vi "2 - 参数计算.vi"(8 "error in (no error)":errorcluster caption="错误输入（无错误）", 10 "采集信号输入":waveform(dbl)[](array[waveform]), 11 "显示控件引用输入":T1) -> (0 "error out":errorcluster caption="错误输出")   [LabVIEW 2019]
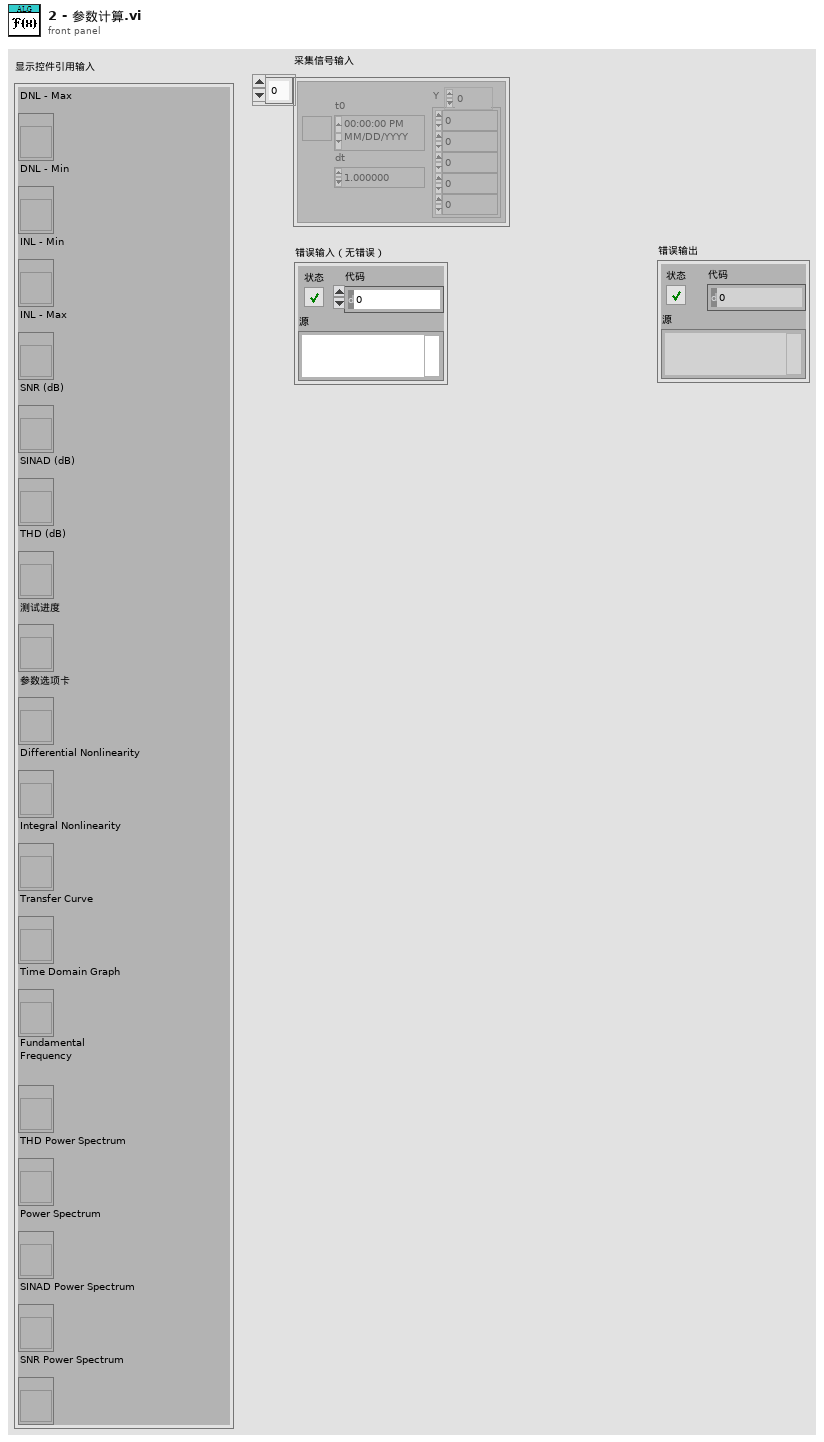
[diagram p1: front panel]
types:
  T1 = cluster{"DNL - Max":refnum<vi>, "DNL - Min":refnum<vi>, "INL - Min":refnum<vi>, "INL - Max":refnum<vi>, "SNR (dB)":refnum<vi>, "SINAD (dB)":refnum<vi>, "THD (dB)":refnum<vi>, "测试进度":refnum<vi>, "参数选项卡":refnum<vi>, "Differential Nonlinearity":refnum<vi>, "Integral Nonlinearity":refnum<vi>, "Transfer Curve":refnum<vi>, "Time Domain Graph":refnum<vi>, "Fundamental\nFrequency":refnum<vi>, "THD Power Spectrum":refnum<vi>, "Power Spectrum":refnum<vi>, "SINAD Power Spectrum":refnum<vi>, "SNR Power Spectrum":refnum<vi>}
  T2 = enum8{"Enabled", "Disabled", "Disabled and Grayed Out"}
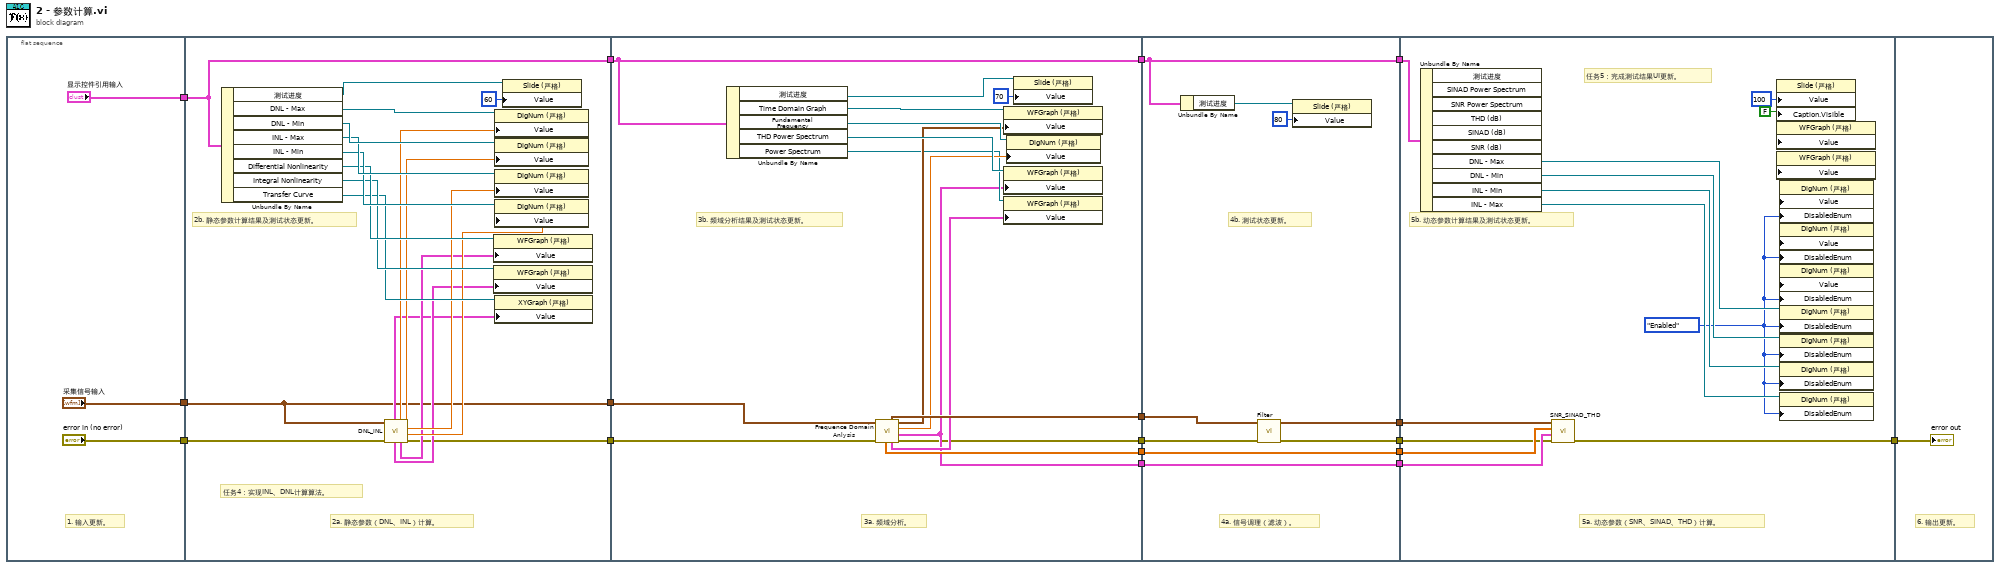
[diagram p0: block diagram]
diagram:
  n1 = flat-sequence {
    tunnel: ["采集信号输入"] -> w17
    tunnel: ["显示控件引用输入"] -> w16
    tunnel: ["error in (no error)"] -> w5
    tunnel: w17 -> [w23]
    tunnel: w16 -> [w24]
    tunnel: [w23] -> w15
    tunnel: [w24] -> w14
    tunnel: w5 -> [w22]
    tunnel: [w21] -> w4
    tunnel: w15 -> [w56]
    tunnel: w14 -> [w46]
    tunnel: [w55] -> w13
    tunnel: [w43] -> w12
    tunnel: [w54] -> w11
    tunnel: [w46] -> w10
    tunnel: w4 -> [w42]
    tunnel: [w41] -> w3
    tunnel: w13 -> [w63]
    tunnel: w12 -> [w65]
    tunnel: w11 -> [w64]
    tunnel: w10 -> [w59]
    tunnel: [w65] -> w9
    tunnel: [w64] -> w8
    tunnel: [w62] -> w7
    tunnel: [w59] -> w6
    tunnel: w3 -> [w58]
    tunnel: [w57] -> w2
    tunnel: w9 -> [w78]
    tunnel: w8 -> [w76]
    tunnel: w7 -> [w77]
    tunnel: w6 -> [w75]
    tunnel: w2 -> [w72]
    tunnel: [w71] -> w1
    tunnel: w1 -> [w79]
    frame #0 {
      # "1. 输入更新。"
    }
    frame #1 {
      # "任务4：实现INL、DNL计算算法。"
      # "2b. 静态参数计算结果及测试状态更新。"
      # "2a. 静态参数（DNL、INL）计算。"
      n2 = Unbundle By Name(w24) -> ("测试进度"=w26:refnum<vi>, "DNL - Max"=w40:refnum<vi>, "DNL - Min"=w39:refnum<vi>, "INL - Max"=w38:refnum<vi>, "INL - Min"=w37:refnum<vi>, "Differential Nonlinearity"=w36:refnum<vi>, "Integral Nonlinearity"=w35:refnum<vi>, "Transfer Curve"=w34:refnum<vi>)
      n3 = call "DNL_INL.vi"("error in (no error)"=w22, "采集信号输入"=w23) -> ("error out"=w21:errorcluster, "INL - Min"=w30:ext, "INL - Max"=w31:ext, "DNL - Min"=w32:dbl, "DNL"=w29:cluster{i32, i32, "Y[i]=X[i]*a+b":dbl[]}, "DNL - Max"=w33:dbl, "INL"=w28:cluster{dbl, i32, ext[]}, "Transfer Curve"=w27:cluster{dbl[], i32[]}[])  [unwired: 2 in]
      n4 = property class="WFGraph (严格)"(reference=w36, "Value"=w29) -> ()  [unwired: 1 in, 2 out]
      n5 = property class="WFGraph (严格)"(reference=w35, "Value"=w28) -> ()  [unwired: 1 in, 2 out]
      n6 = property class="DigNum (严格)"(reference=w40, "Value"=w33) -> ()  [unwired: 1 in, 2 out]
      n7 = property class="DigNum (严格)"(reference=w39, "Value"=w32) -> ()  [unwired: 1 in, 2 out]
      n8 = property class="DigNum (严格)"(reference=w38, "Value"=w31) -> ()  [unwired: 1 in, 2 out]
      n9 = property class="DigNum (严格)"(reference=w37, "Value"=w30) -> ()  [unwired: 1 in, 2 out]
      n10 = property class="XYGraph (严格)"(reference=w34, "Value"=w27) -> ()  [unwired: 1 in, 2 out]
      n11 = property class="Slide (严格)"(reference=w26, "Value"=u8 60 ("值")) -> ()  [unwired: 1 in, 2 out]
    }
    frame #2 {
      # "3b. 频域分析结果及测试状态更新。"
      # "3a. 频域分析。"
      n12 = Unbundle By Name(w46) -> ("测试进度"=w53:refnum<vi>, "Time Domain Graph"=w51:refnum<vi>, "Fundamental\nFrequency"=w50:refnum<vi>, "THD Power Spectrum"=w49:refnum<vi>, "Power Spectrum"=w45:refnum<vi>)
      n13 = call "Frequence Domain Anlysis.vi"("error in (no error)"=w42, "采集信号输入"=w56) -> ("error out"=w41:errorcluster, "THD Power Spectrum"=w43:cluster{"f0":dbl, "df":dbl, "magnitude":dbl[]}[], "detected fundamental frequency"=w47:dbl, "S-Waveform Out"=w48:waveform(dbl), "power spectrum"=w44:cluster{"f0":dbl, "df":dbl, "magnitude":dbl[]}, "O-Waveform"=w55:waveform(dbl), "Harmonics Data Out"=w54:dbl[])  [unwired: 3 in]
      n14 = property class="WFGraph (严格)"(reference=w51, "Value"=w48) -> ()  [unwired: 1 in, 2 out]
      n15 = property class="WFGraph (严格)"(reference=w49, "Value"=w43) -> ()  [unwired: 1 in, 2 out]
      n16 = property class="WFGraph (严格)"(reference=w45, "Value"=w44) -> ()  [unwired: 1 in, 2 out]
      n17 = property class="DigNum (严格)"(reference=w50, "Value"=w47) -> ()  [unwired: 1 in, 2 out]
      n18 = property class="Slide (严格)"(reference=w53, "Value"=u8 70 ("值")) -> ()  [unwired: 1 in, 2 out]
    }
    frame #3 {
      # "4b. 测试状态更新。"
      # "4a. 信号调理（滤波）。"
      n19 = Unbundle By Name(w59) -> ("测试进度"=w61:refnum<vi>)
      n20 = call "Filter.vi"("error in (no error)"=w58, "O-Waveform输入"=w63) -> ("error out"=w57:errorcluster, "F_Waveform输出"=w62:waveform(dbl))  [unwired: 8 in]
      n21 = property class="Slide (严格)"(reference=w61, "Value"=u8 80 ("值")) -> ()  [unwired: 1 in, 2 out]
    }
    frame #4 {
      w66 = T2."Enabled" ("禁用")
      # "任务5：完成测试结果UI更新。"
      # "5b. 动态参数计算结果及测试状态更新。"
      # "5a. 动态参数（SNR、SINAD、THD）计算。"
      n22 = Unbundle By Name(w75) -> ("DNL - Max"=w67:refnum<vi>, "DNL - Min"=w68:refnum<vi>, "INL - Min"=w69:refnum<vi>, "INL - Max"=w70:refnum<vi>)  [unwired: 6 out]
      n23 = call "SNR_SINAD_THD.vi"("error in (no error)"=w72, "THD Power Spectrum"=w78, "Harmonics Data Out"=w76, "F_Waveform输入"=w77) -> ("error out"=w71:errorcluster)  [unwired: 2 in, 5 out]
      n24 = property class="Slide (严格)"("Value"=u8 100 ("值"), "Caption.Visible"=FALSE ("标题.可见")) -> ()  [unwired: 2 in, 2 out]
      n25 = property class="WFGraph (严格)" props=["Value"]() -> ()  [unwired: 3 in, 2 out]
      n26 = property class="WFGraph (严格)" props=["Value"]() -> ()  [unwired: 3 in, 2 out]
      n27 = property class="DigNum (严格)" props=["Value", "DisabledEnum"]("DisabledEnum"=w66) -> ()  [unwired: 3 in, 2 out]
      n28 = property class="DigNum (严格)" props=["Value", "DisabledEnum"]("DisabledEnum"=w66) -> ()  [unwired: 3 in, 2 out]
      n29 = property class="DigNum (严格)" props=["Value", "DisabledEnum"]("DisabledEnum"=w66) -> ()  [unwired: 3 in, 2 out]
      n30 = property class="DigNum (严格)"(reference=w67, "DisabledEnum"=w66) -> ()  [unwired: 1 in, 2 out]
      n31 = property class="DigNum (严格)"(reference=w68, "DisabledEnum"=w66) -> ()  [unwired: 1 in, 2 out]
      n32 = property class="DigNum (严格)"(reference=w69, "DisabledEnum"=w66) -> ()  [unwired: 1 in, 2 out]
      n33 = property class="DigNum (严格)"(reference=w70, "DisabledEnum"=w66) -> ()  [unwired: 1 in, 2 out]
    }
    frame #5 {
      # "6. 输出更新。"
      "error out" <- w79
    }
  }
